vi "读取矩阵温度.vi"(0 "x1":u16, 5 "y1":u16, 7 "x2":u16, 9 "y2":u16, 11 "error in":errorcluster) -> (8 "温度":dbl, 15 "error out":errorcluster)   [LabVIEW 2016]
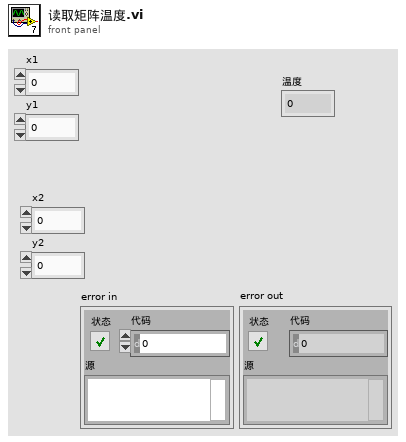
[diagram p1: front panel]
types:
  T1 = cluster{"byCmdType":u8, "bySubCmd":u8, "byParam_h":u8, "byParam_l":u8, "byAddr1_hh":u8, "byAddr1_h":u8, "byAddr1_l":u8, "byAddr1_ll":u8, "byAddr2_hh":u8, "byAddr2_h":u8, "byAddr2_l":u8, "byAddr2_ll":u8, "byLen_hh":u8, "byLen_h":u8, "byLen_l":u8, "byLen_ll":u8}
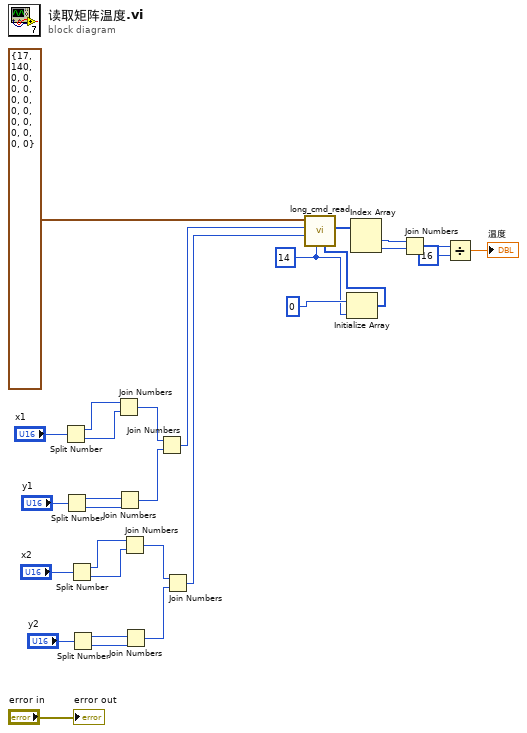
[diagram p0: block diagram]
diagram:
  w2 = u32 14 ("dwLen")
  n1 = Split Number(x="x1") -> (hi(x)=w26:u8, lo(x)=w25:u8)
  n2 = Split Number(x="y1") -> (hi(x)=w24:u8, lo(x)=w23:u8)
  n3 = Split Number(x="x2") -> (hi(x)=w8:u8, lo(x)=w9:u8)
  n4 = Split Number(x="y2") -> (hi(x)=w10:u8, lo(x)=w11:u8)
  n5 = Join Numbers(hi=w26, lo=w25) -> ((hi.lo)=w21:u16)
  n6 = Join Numbers(hi=w24, lo=w23) -> ((hi.lo)=w22:u16)
  n7 = Join Numbers(hi=w8, lo=w9) -> ((hi.lo)=w13:u16)
  n8 = Join Numbers(hi=w10, lo=w11) -> ((hi.lo)=w12:u16)
  n9 = Join Numbers(hi=w21, lo=w22) -> ((hi.lo)=w20:u32)
  n10 = Join Numbers(hi=w13, lo=w12) -> ((hi.lo)=w5:u32)
  n11 = Initialize Array(u32 0 ("dwLen"), w2) -> (w1:u32[])
  n12 = call "long_cmd_read.vi"("data"=w1, "dwLen"=w2, "dwAddr2"=w5, "dwAddr1"=w20, "vd_cmd_long_header_t"=T1 {"byCmdType"=17, "bySubCmd"=140, "byParam_h"=0, "byParam_l"=0, "byAddr1_hh"=0, "byAddr1_h"=0, "byAddr1_l"=0, "byAddr1_ll"=0, "byAddr2_hh"=0, "byAddr2_h"=0, "byAddr2_l"=0, "byAddr2_ll"=0, "byLen_hh"=0, "byLen_h"=0, "byLen_l"=0, "byLen_ll"=0}) -> ("data out"=w19:u8[])  [unwired: 4 in, 2 out]
  n13 = Index Array(array=w19) -> (element #1=w18:u8, element #2=w17:u8)  [unwired: 2 in]
  n14 = Join Numbers(hi=w18, lo=w17) -> ((hi.lo)=w16:u16)
  n15 = Divide(x=w16, y=u16 16) -> (x/y=→"温度":dbl)
  "error out" <- "error in"
